vi "ToString.vi"(11 "Journal In":refnum<class "Journal.lvclass">) -> (2 "String":string, 3 "Journal Out":refnum<class "Journal.lvclass">)   [LabVIEW 2018, in "Journal.lvclass"]
uses:
  Journal.lvclass
  Journal.lvclass/Journal.ctl
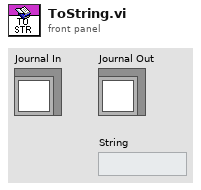
[diagram p1: front panel]
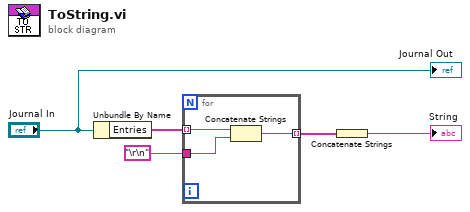
[diagram p0: block diagram]
diagram:
  n1 = Unbundle By Name("Journal In") -> ("Entries"=w4:string[])
  n2 = for {
    tunnel: w4 -> [w8] mode=indexing
    tunnel: "\r\n" -> [w7]
    tunnel: [w6] -> w2 mode=indexing
    n3 = Concatenate Strings(w8, w7) -> (w6:string)
  }
  n4 = Concatenate Strings(w2) -> (→"String":string)
  "Journal Out" <- "Journal In"
